vi "R_S_waitingTime.vi"(7 "Waiting Time(ms)":u32=1000, 8 "error in":errorcluster) -> (0 "error out":errorcluster)   [LabVIEW 2023, in "R_S.lvlib"]
uses:
  R_S.lvlib
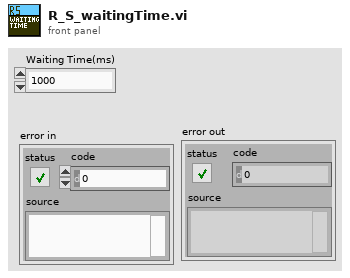
[diagram p1: front panel]
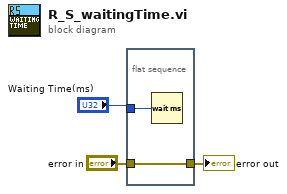
[diagram p0: block diagram]
diagram:
  n1 = flat-sequence {
    tunnel: "error in" -> [w5]
    tunnel: [w5] -> w2
    tunnel: "Waiting Time(ms)" -> [w4]
    frame #0 {
      n2 = Wait (ms)(milliseconds to wait=w4) -> ()  [unwired: 1 out]
    }
  }
  "error out" <- w2
